vi "FTW-Tree-PointToItem.vi"(0 "Tree Ctl Ref":refnum<vi>, 5 "Coords":cluster{"Left":i32, "Top":i32}, 11 "error in":errorcluster) -> (4 "Tree Ctl Ref out":refnum<vi>, 6 "Tag":string, 8 "Column":i32, 15 "error out":errorcluster)   [LabVIEW 2012]
panel:
  # "Inputs"
  # "Outputs"
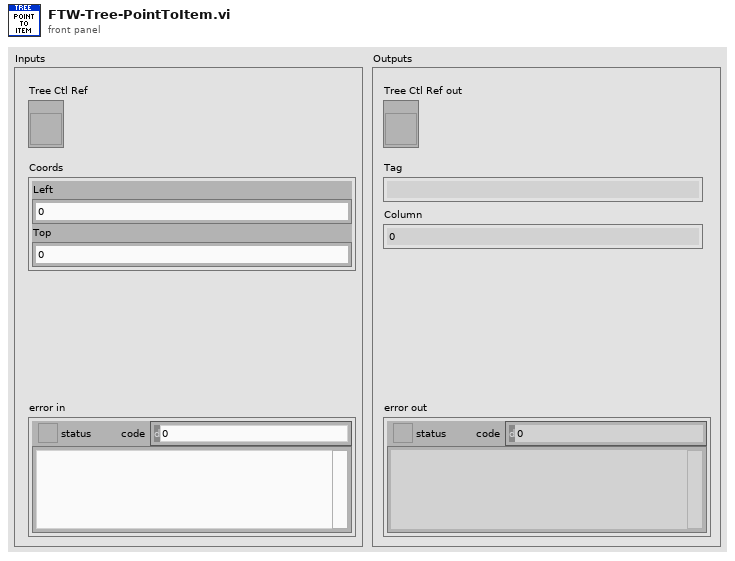
[diagram p1: front panel]
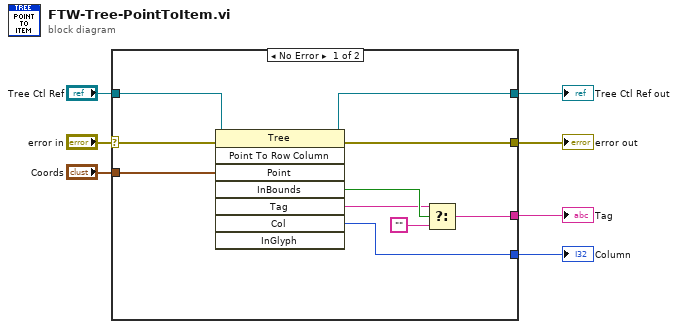
[diagram p0: block diagram]
diagram:
  n1 = case shown="No Error" "error in" {
    selector: "error in" -> [w17 w19]
    tunnel: [w16 w19] -> w7
    tunnel: "Tree Ctl Ref" -> [w10 w18]
    tunnel: "Coords" -> [w8 _]
    tunnel: [w11 _] -> w3
    tunnel: [w14 _] -> w2
    tunnel: [w9 w18] -> w1
    frame No Error {
      n2 = invoke on="Invoke Node" class="Tree" method="Point To Row Column"(reference=w10, error in=w17, "Point"=w8) -> (reference out=w9:refnum<vi>, error out=w16:errorcluster, "InBounds"=w13:bool, "Tag"=w12:string, "Col"=w11:i32)  [unwired: 5 in, 3 out]
      n3 = Select(t=w12, s=w13, f="") -> (s? t:f=w14:string)
    }
    frame Error {
    }
  }
  "error out" <- w7
  "Tag" <- w2
  "Column" <- w3
  "Tree Ctl Ref out" <- w1
